vi "Handle Last Ack Core.vi"(4 "error in (no error)":errorcluster, 6 "Last Ack":refnum<class "Last Ack.lvclass">, 7 "OPC Server in":refnum<class "OPC Server.lvclass">) -> (0 "error out":errorcluster, 3 "OPC Server out":refnum<class "OPC Server.lvclass">)   [LabVIEW 2021, in "OPC Server.lvlib" / "OPC Server.lvclass"]
doc: "(<B>Filename</B>: Actor Framework.lvlib:Actor.lvclass:Handle Last Ack Core.vi)\n\nDefines how the caller actor responds to the Last Ack message from a nested actor. The Last Ack message is the final message a nested actor sends to its caller before it shuts down. The message contains information about the final state of the nested actor.\n\nBy default, this method does nothing except return any error the nested actor sent. A descendant class may override this method to define behavior."
uses:
  OPC Server.lvclass
  <vilib>/ActorFramework/LastAck/Last Ack.lvclass
  OPC Server.lvclass/OPC Server.ctl
  <vilib>/ActorFramework/Actor/Actor.lvclass
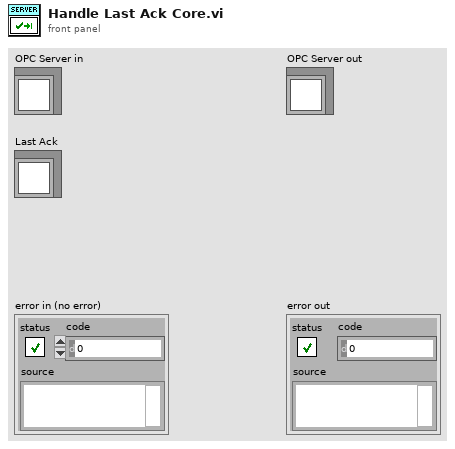
[diagram p1: front panel]
types:
  T1 = map{string, refnum<class "Message Enqueuer.lvclass">}
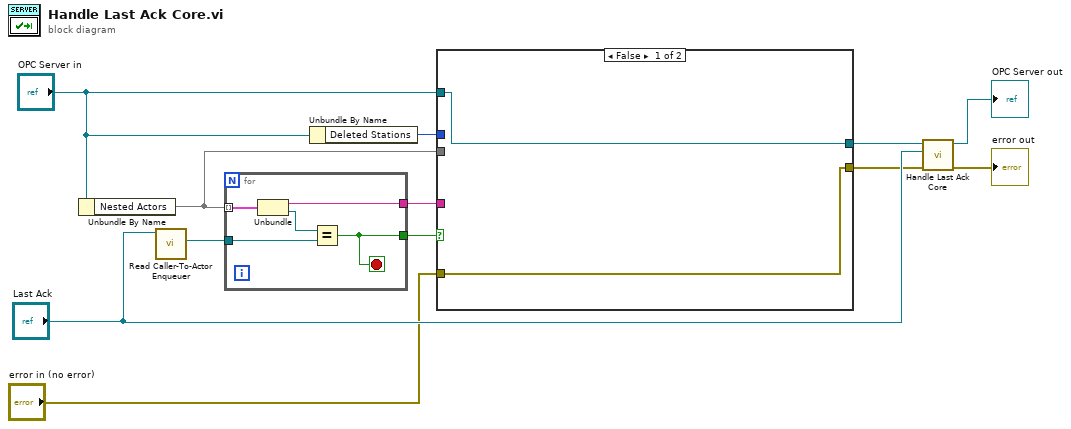
[diagram p0: block diagram]
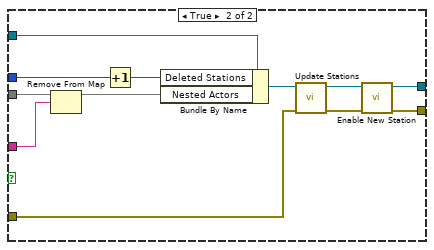
[diagram p2: hidden frame]
diagram:
  n1 = Unbundle By Name("OPC Server in") -> ("Nested Actors"=w7:T1)
  n2 = call <vilib>:"Read Caller-To-Actor Enqueuer.vi"("Last Ack"="Last Ack") -> ("Caller-to-Actor Enqueuer"=w9:refnum<class "Message Enqueuer.lvclass">)  [unwired: 10 in]
  n3 = for {
    tunnel: w7 -> [w17] mode=indexing
    tunnel: w9 -> [w16]
    tunnel: [w14] -> w6
    tunnel: [w13] -> w5
    stop <- w14 stop-if-true
    n4 = Unbundle(w17) -> (w13:string, "Enqueuer"=w15:refnum<class "Message Enqueuer.lvclass">)
    n5 = Equal?(x=w15, y=w16) -> (x = y?=w14:bool)
  }
  n6 = Unbundle By Name("OPC Server in") -> ("Deleted Stations"=w3:u32)
  n7 = case shown="False" w6 {
    tunnel: "OPC Server in" -> [w19 w27]
    tunnel: w7 -> [_ w31]
    tunnel: w5 -> [_ w30]
    tunnel: [w19 w23] -> w4
    tunnel: w3 -> [_ w26]
    tunnel: "error in (no error)" -> [w18 w21]
    tunnel: [w18 w20] -> w1
    frame False {
    }
    frame True {
      n8 = Remove From Map(10:w30, 11:w31) -> (3:w29:T1)  [unwired: 2 out]
      n9 = Increment(x=w26) -> (x+1=w25:u32)
      n10 = Bundle By Name(cluster=w27, "Deleted Stations"=w25, "Nested Actors"=w29) -> (w28:refnum<class "OPC Server.lvclass">)
      n11 = call "Update Stations.vi"("error in (no error)"=w21, "OPC Server in"=w28) -> ("error out"=w22:errorcluster, "OPC Server out"=w24:refnum<class "OPC Server.lvclass">)  [unwired: 8 in]
      n12 = call "Enable New Station.vi"("error in (no error)"=w22, "OPC Server in"=w24) -> ("error out"=w20:errorcluster, "OPC Server out"=w23:refnum<class "OPC Server.lvclass">)  [unwired: 8 in]
    }
  }
  n13 = call-parent "Handle Last Ack Core.vi"("error in (no error)"=w1, "Last Ack"="Last Ack", "Actor in"=w4) -> ("error out"=→"error out":errorcluster, "Actor out"=→"OPC Server out":refnum<class "OPC Server.lvclass">)  [unwired: 3 in]
